vi "Case.vi"() -> ()   [LabVIEW 2021]
panel:
  out "Numeric 2":dbl
  in  "Numeric":dbl
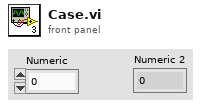
[diagram p1: front panel]
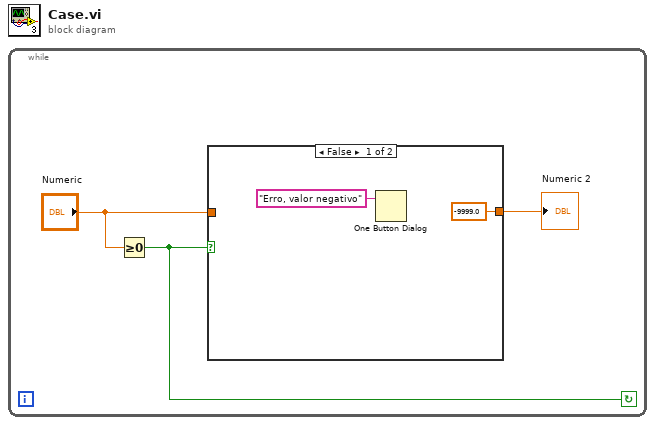
[diagram p0: block diagram]
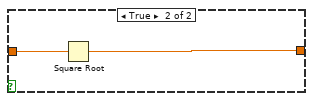
[diagram p2: hidden frame]
diagram:
  n1 = while {
    stop <- w1 continue-if-true
    n2 = Greater Or Equal To 0?(x="Numeric") -> (x >= 0?=w1:bool)
    n3 = case shown="False" w1 {
      tunnel: "Numeric" -> [_ w7]
      tunnel: [-9999.0 w6] -> w2
      frame False {
        n4 = One Button Dialog(message="Erro, valor negativo") -> ()  [unwired: 1 in, 1 out]
      }
      frame True {
        n5 = Square Root(x=w7) -> (sqrt(x)=w6:dbl)
      }
    }
    "Numeric 2" <- w2
  }
